vi "LINE_1.vi"() -> ()   [LabVIEW 2019]
panel:
  in  "LINE_1_in":string
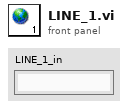
[diagram p1: front panel]
diagram:
